vi "Write Value.vi"(8 "error in (no error)":errorcluster, 10 "Data":T1, 11 "Numeric in":refnum<class "Const_Time.lvclass">) -> (0 "error out":errorcluster, 3 "Numeric out":refnum<class "Const_Time.lvclass">)   [LabVIEW 2021, in "Const_Time.lvclass"]
uses:
  Const_Time.lvclass
  Type.ctl
  Const_Time.lvclass/Const_Time.ctl
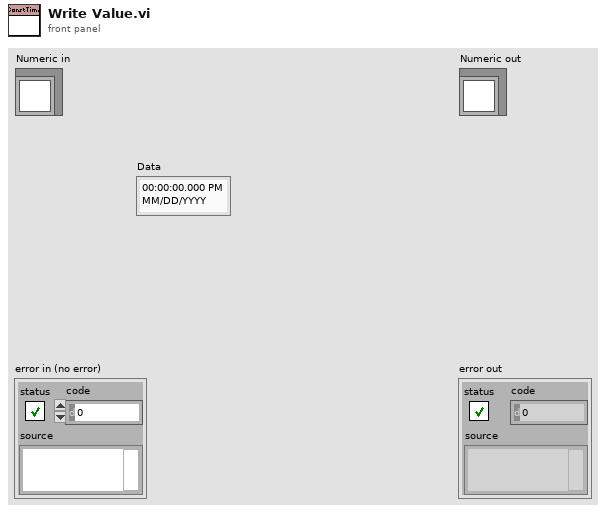
[diagram p1: front panel]
types:
  T1 = typedef "Const_Time.lvclass/Type.ctl" = timestamp
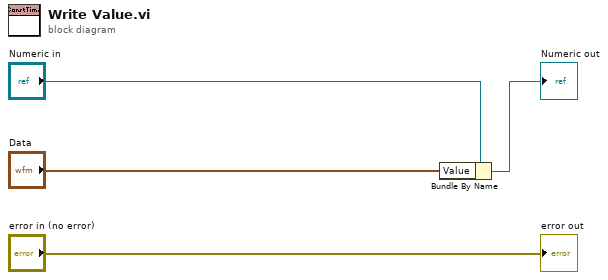
[diagram p0: block diagram]
diagram:
  n1 = Bundle By Name(cluster="Numeric in", "Value"="Data") -> (→"Numeric out":refnum<class "Const_Time.lvclass">)
  "error out" <- "error in (no error)"
